vi "Cmd-Reply.vi"(8 "error in (no error)":errorcluster, 9 "ms to wait":u32=200, 10 "cmd":string="s", 11 "VISA Refnum in":refnum<visa-resource-name>="COM1") -> (0 "error out":errorcluster={"status"=FALSE, "code"=1073676294, "source"="VISA Read in Cmd-Reply.vi"}, 1 "reply":string="\r\nstandby        ", 3 "VISA Refnum out":refnum<visa-resource-name>="COM1")   [LabVIEW 2022 SP3]
uses:
  <vilib>/Utility/error.llb/Trim Whitespace One-Sided.vi
panel:
  out "read buffer":string
  out "Write return count":u32=4
  out "Bytes at Serial Port":u32=17
  # "1073676294 is normal\nwarning that last char\nread might not be last \nchar in buffer.\n\nwith initial /r/n and \nno termination char,\nread #bytes in buffer, this\nis to be expected."
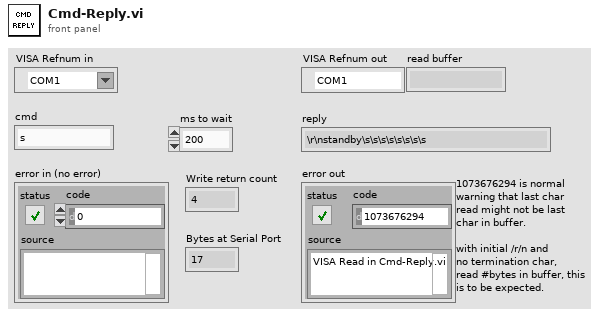
[diagram p1: front panel]
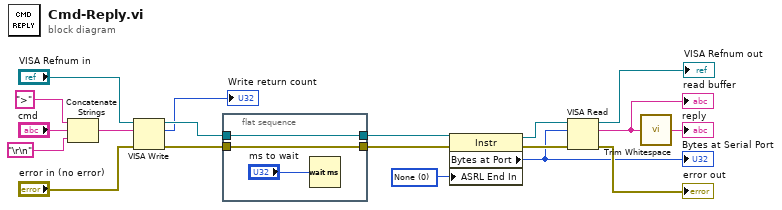
[diagram p0: block diagram]
diagram:
  w3 = u16 0 items=["None", "Last Bit", "TermChar"] ("Serial Settings:End Mode for Reads")
  n1 = Concatenate Strings(">" ("string"), "cmd", "\r\n") -> (w9:string)
  n2 = VISA Write(VISA resource name="VISA Refnum in", write buffer=w9, error in (no error)="error in (no error)") -> (VISA resource name out=w11:refnum<visa-resource-name>, return count=→"Write return count":u32, error out=w13:errorcluster)
  n3 = flat-sequence {
    tunnel: w13 -> [w21]
    tunnel: [w21] -> w12
    tunnel: w11 -> [w20]
    tunnel: [w20] -> w10
    frame #0 {
      n4 = Wait (ms)(milliseconds to wait="ms to wait") -> ()  [unwired: 1 out]
    }
  }
  n5 = property class="Instr"(reference=w10, error in=w12, "ASRL End In"=w3) -> (reference out=w15:refnum<visa-resource-name>, error out=w14:errorcluster, "Bytes at Port"=w4:u32)
  "Bytes at Serial Port" <- w4
  n6 = VISA Read(VISA resource name=w15, byte count=w4, error in (no error)=w14) -> (VISA resource name out=→"VISA Refnum out":refnum<visa-resource-name>, read buffer=w2:string, error out=→"error out":errorcluster)  [unwired: 1 out]
  "read buffer" <- w2
  n7 = call <vilib>:"Trim Whitespace.vi"("string"=w2) -> ("trimmed string"=→"reply":string)  [unwired: 1 in]
